vi "Arrays Count How High.vi"() -> ()   [LabVIEW 2019]
panel:
  out "Count":i32[](array[numeric])
  in  "How High?":i32
  # "Challenge:\nCount from 1 to a specified integer between 1 and 20."
  # "Try it: Enter an integer between 1 and 20 in the \"How High?\" box and hit Run."
  # "You will probably need:\nArrays, for loops, numeric functions"
  # "Open the block diagram to see a possible solution."
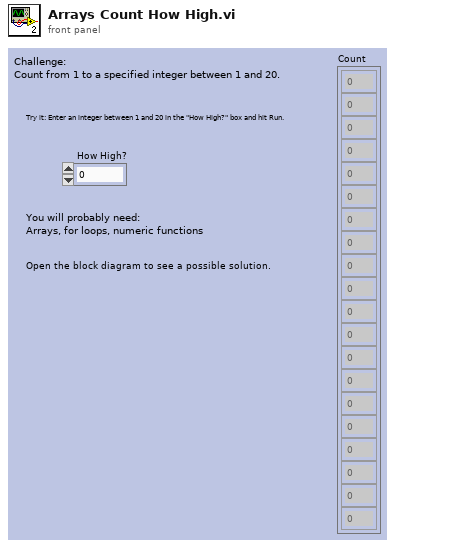
[diagram p1: front panel]
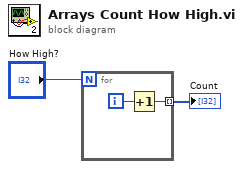
[diagram p0: block diagram]
diagram:
  n1 = for {
    N: "How High?" -> [_]
    tunnel: [w3] -> w1 mode=indexing
    i -> [w4]
    n2 = Increment(x=w4) -> (x+1=w3:i32)
  }
  "Count" <- w1
